vi "Experiment header-Read keys.vi"(8 "error in (no error)":errorcluster, 10 "All Parameter names":T1[](array[typedef]), 11 "FIle refnum IN":T2) -> (0 "error out":errorcluster, 3 "FIle refnum OUT":T2)   [LabVIEW 2017]
uses:
  <vilib>/Utility/config.llb/Config Data RefNum.ctl
  Typedefs/Header file parameter names.ctl
  <vilib>/Utility/config.llb/NI_LVConfig.lvlib
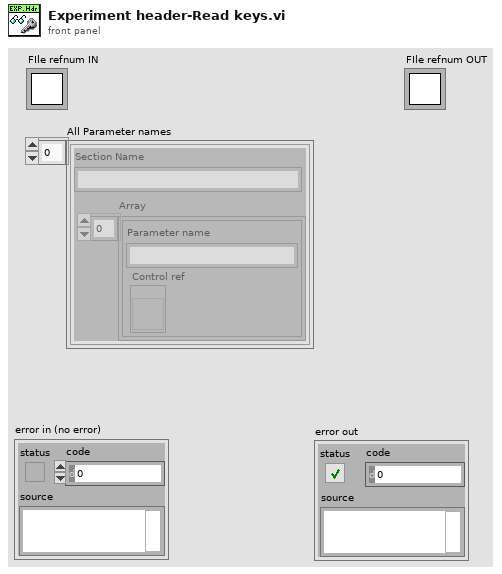
[diagram p1: front panel]
types:
  T1 = typedef "Header file parameter names.ctl" = cluster{"Section Name":string, "Array":cluster{"Parameter name":string, "Control ref":refnum<vi>}[]}
  T2 = typedef "NI_LVConfig.lvlib/Config Data RefNum.ctl" = refnum<k1>
  T3 = cluster{"Parameter name":string, "Control ref":refnum<vi>}[]
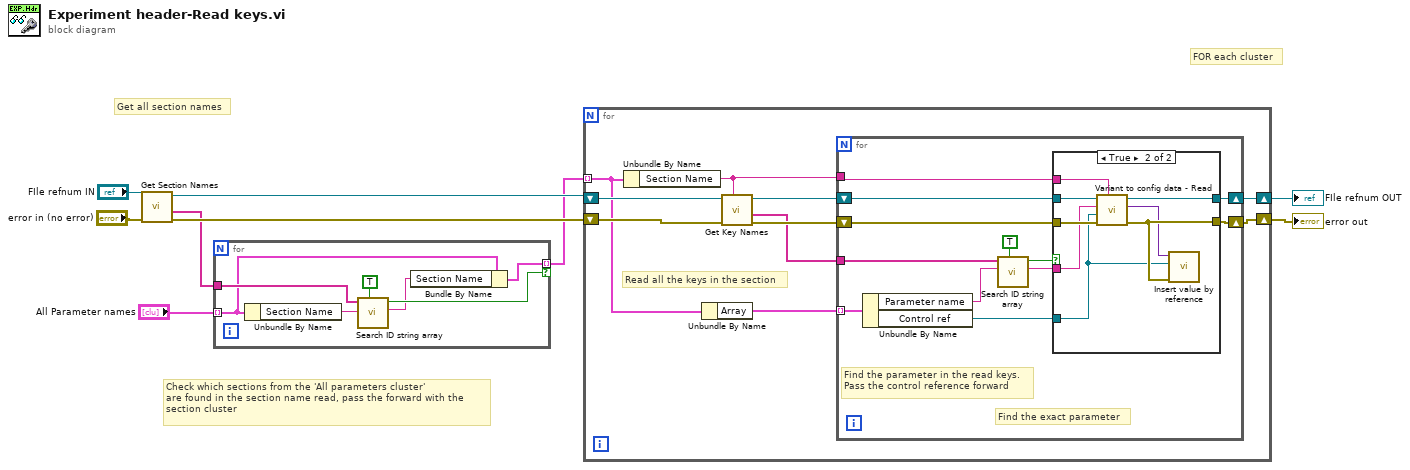
[diagram p0: block diagram]
diagram:
  # "FOR each cluster"
  # "Check which sections from the 'All parameters cluster'\nare found in the section name read, pass the forward with the\nsection cluster"
  # "Get all section names"
  n1 = call <vilib>:"Get Section Names.vi"("error in (no error)"="error in (no error)", "refnum"="FIle refnum IN") -> ("error out"=w6:errorcluster, "section names"=w3:string[], "refnum out"=w7:T2)  [unwired: 7 in]
  n2 = for {
    tunnel: w3 -> [w16]
    tunnel: "All Parameter names" -> [w13] mode=indexing
    tunnel: [w11] -> w4 mode=indexing if=w14
    n3 = Unbundle By Name(w13) -> ("Section Name"=w15:string)
    n4 = call "Search ID string array.vi"("With lower case ?"=TRUE, "Input String"=w15, "String Array"=w16) -> ("Match String"=w12:string, "String found ?"=w14:bool)  [unwired: 7 in]
    n5 = Bundle By Name(cluster=w13, "Section Name"=w12) -> (w11:T1)
  }
  n6 = for {
    shift-right: [w18] -> w2
    shift-left: w7 -> [w26]
    shift-right: [w17] -> w1
    shift-left: w6 -> [w25]
    tunnel: w4 -> [w24] mode=indexing
    # "Read all the keys in the section"
    n7 = Unbundle By Name(w24) -> ("Section Name"=w21:string)
    n8 = Unbundle By Name(w24) -> ("Array"=w23:T3)
    n9 = call <vilib>:"Get Key Names.vi"("section"=w21, "error in (no error)"=w25, "refnum"=w26) -> ("error out"=w20:errorcluster, "key names"=w19:string[], "refnum out"=w22:T2)  [unwired: 5 in, 1 out]
    n10 = for {
      tunnel: w19 -> [w35]
      tunnel: w23 -> [w38] mode=indexing
      shift-right: [w28] -> w18
      shift-left: w22 -> [w37]
      tunnel: w21 -> [w29]
      shift-right: [w27] -> w17
      shift-left: w20 -> [w36]
      # "Find the exact parameter"
      # "Find the parameter in the read keys.\nPass the control reference forward"
      n11 = Unbundle By Name(w38) -> ("Parameter name"=w33:string, "Control ref"=w31:refnum<vi>)
      n12 = call "Search ID string array.vi"("With lower case ?"=TRUE, "Input String"=w33, "String Array"=w35) -> ("Match String"=w30:string, "String found ?"=w32:bool)  [unwired: 7 in]
      n13 = case shown="True" w32 {
        tunnel: w37 -> [w39 w48]
        tunnel: w36 -> [w40 w47]
        tunnel: w31 -> [_ w41]
        tunnel: w30 -> [_ w46]
        tunnel: w29 -> [_ w45]
        tunnel: [w39 w44] -> w28
        tunnel: [w40 w43] -> w27
        frame False {
        }
        frame True {
          n14 = call "Variant to config data - Read.vi"("Section Name"=w45, "error in (no error)"=w47, "Control in"=w41, "Key Name"=w46, "FIle refnum IN"=w48) -> ("error out"=w43:errorcluster, "Value"=w42:variant, "Refnum out"=w44:T2)  [unwired: 4 in]
          n15 = call "Insert value by reference.vi"("error in (no error)"=w43, "Control in"=w41, "Variant value IN"=w42) -> ()  [unwired: 8 in, 1 out]
        }
      }
    }
  }
  "FIle refnum OUT" <- w2
  "error out" <- w1
